vi "NTJ_OldVer_GetFieldData.vi"(7 "error in (no error)":errorcluster, 10 "Entry Name":string) -> (0 "error out":errorcluster, 2 "Field Value Out":T2, 3 "Entry ID":T1)   [LabVIEW 2019]
uses:
  <vilib>/Rock Robotics/Network Tables/Field Data.ctl
  <vilib>/Rock Robotics/Network Tables/Field Type.ctl
  <vilib>/Rock Robotics/Network Tables/Sequence.ctl
  <vilib>/Rock Robotics/Network Tables/Field ID.ctl
  <vilib>/Rock Robotics/Network Tables/Create Actual Table Name.vi
  <vilib>/Rock Robotics/Network Tables/NT Globals.vi
  <vilib>/Rock Robotics/Network Tables/Table Manager.vi
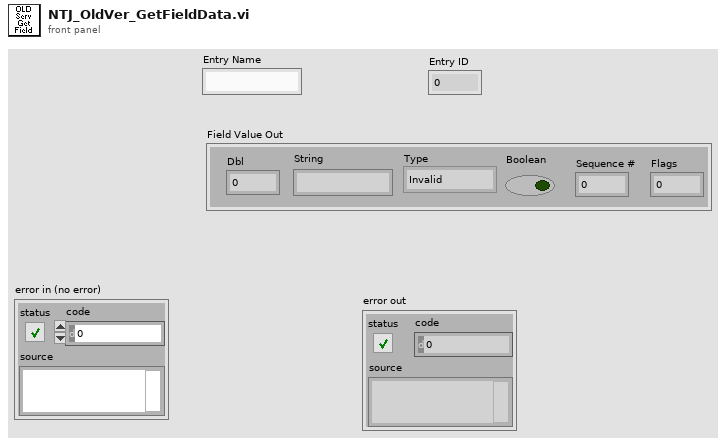
[diagram p1: front panel]
types:
  T1 = typedef "Field ID.ctl" = i32
  T2 = typedef "Field Data.ctl" = cluster{"Dbl":dbl, "String":string, "Type":T3, "Boolean":bool, "Sequence #":T4, "Flags":u8}
  T3 = typedef "Field Type.ctl" = enum8{"Invalid", "Bool", "Numeric", "String", "Raw", "Boolean Array", "Numeric Array", "String Array", "RPC"}
  T4 = typedef "Sequence.ctl" = u16
  T5 = enum16{"Update Field", "Read Field", "Assign Field", "Remove All", "Set Persistence", "Clear Persistence"}
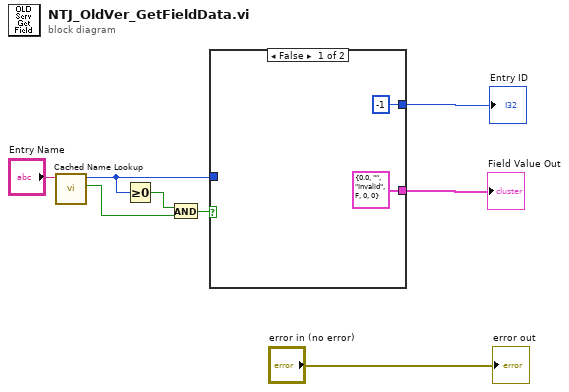
[diagram p0: block diagram]
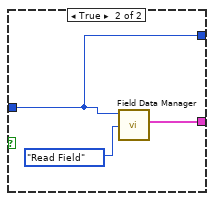
[diagram p2: hidden frame]
diagram:
  n1 = call <vilib>:"Cached Name Lookup.vi"("Name"="Entry Name") -> ("Success"=w3:bool, "Entry ID"=w8:T1)  [unwired: 8 in, 1 out]
  n2 = Greater Or Equal To 0?(x=w8) -> (x >= 0?=w2:bool)
  n3 = And(x=w2, y=w3) -> (x .and. y?=w4:bool)
  n4 = case shown="False" w4 {
    tunnel: w8 -> [_ w11]
    tunnel: [T2 {"Dbl"=0.0, "String"="", "Type"=enum."Invalid", "Boolean"=FALSE, "Sequence #"=0, "Flags"=0} ("Field Value Out") w12] -> w5
    tunnel: [T1 -1 ("Entry ID") w11] -> w1
    frame False {
    }
    frame True {
      n5 = call <vilib>:"Field Data Manager.vi"("Operation"=T5."Read Field", "Field ID"=w11) -> ("Field Value Out"=w12:T2)  [unwired: 8 in, 1 out]
    }
  }
  "Field Value Out" <- w5
  "Entry ID" <- w1
  "error out" <- "error in (no error)"
